vi "Rotating Ring.vi"(8 "error in (no error)":errorcluster, 11 "[V] Login in":refnum<class "[V] Login.lvclass">) -> (0 "error out":errorcluster, 3 "[V] Login out":refnum<class "[V] Login.lvclass">)   [LabVIEW 2020, in "[V] Login.lvlib" / "[V] Login.lvclass"]
uses:
  [V] Login.lvclass
  <vilib>/Analysis/NI_AALBase.lvlib
  <vilib>/Analysis/1siggen.llb/Ramp Pattern by Samples.vi
  <vilib>/picture/picture.llb/Draw True-Color Pixmap.vi
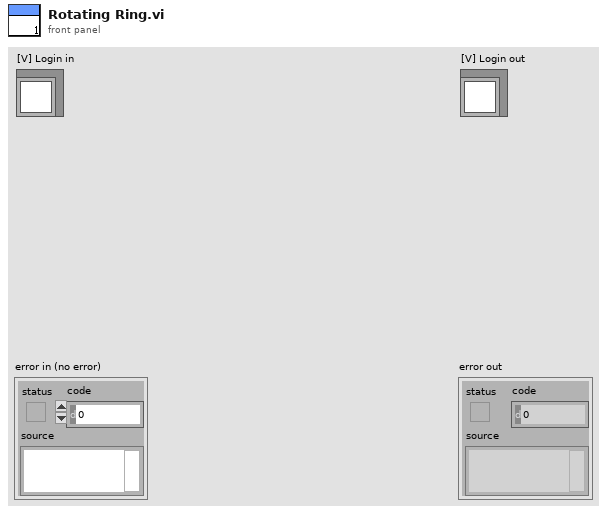
[diagram p1: front panel]
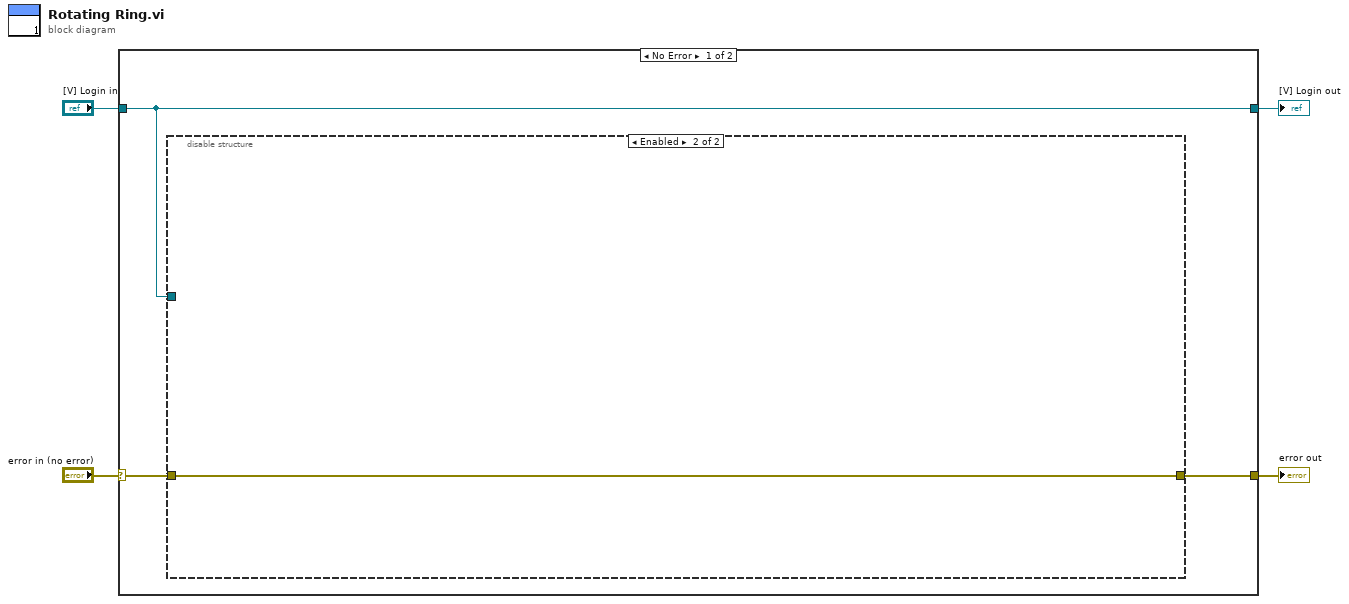
[diagram p0: block diagram]
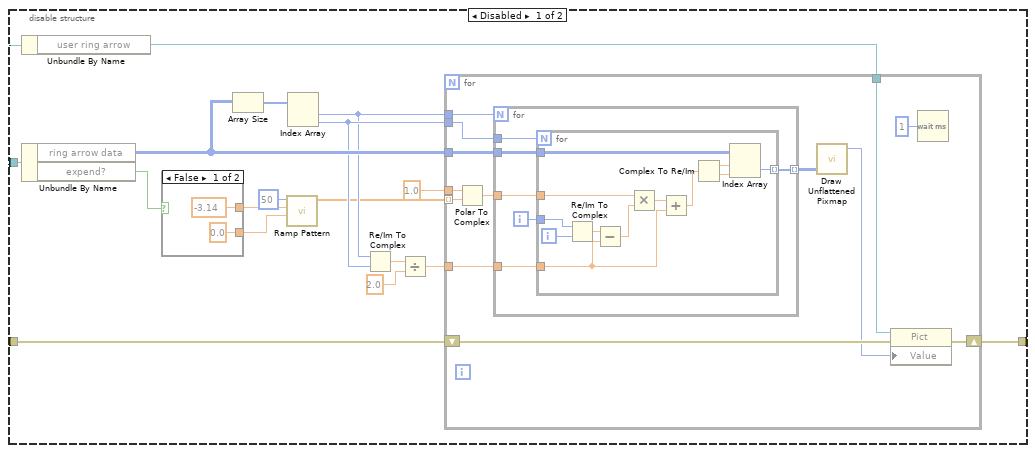
[diagram p2: hidden frame]
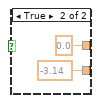
[diagram p3: hidden frame]
diagram:
  n1 = case shown="No Error" "error in (no error)" {
    selector: "error in (no error)" -> [w7 w62]
    tunnel: [w6 w62] -> w3
    tunnel: [w5 w61] -> w1
    tunnel: "[V] Login in" -> [w5 w61]
    frame No Error {
      n2 = disable-structure shown="Enabled" {
        disable-tunnel: w7 -> [w19 w60]
        disable-tunnel: [w16 w60] -> w6
        disable-tunnel: w5 -> [w8 _]
        frame Disabled {
          n3 = Unbundle By Name(w8) -> ("user ring arrow"=w18:refnum<vi>)
          n4 = Unbundle By Name(w8) -> ("ring arrow data"=w21:u32[][], "expend?"=w14:bool)
          n5 = case shown="False" w14 {
            tunnel: [-3.14 ("t") 0.0 ("t")] -> w13
            tunnel: [0.0 ("t") -3.14 ("t")] -> w10
            frame False {
            }
            frame True {
            }
          }
          n6 = Array Size(array=w21) -> (size(s)=w23:i32[])
          n7 = call-poly <vilib>:"Ramp Pattern.vi"("start"=w10, "end"=w13, "samples"=50) -> ("Ramp Pattern"=w11:dbl[])  [unwired: 7 in, 1 out]
          n8 = Index Array(array=w23) -> (element #1=w15:i32, element #2=w17:i32)  [unwired: 2 in]
          n9 = Re/Im To Complex(1:w17, 2:w15) -> (0:w24:cdb)
          n10 = Divide(x=w24, y=2.0) -> (x/y=w20:cdb)
          n11 = for {
            tunnel: w21 -> [w40]
            tunnel: w20 -> [w39]
            shift-right: [w36] -> w16
            shift-left: w19 -> [w37]
            tunnel: w18 -> [w35]
            tunnel: w17 -> [w33]
            tunnel: w11 -> [w32] mode=indexing
            tunnel: w15 -> [w31]
            tunnel: 1.0 ("r") -> [w30]
            n12 = Polar To Complex(1:w32, 2:w30) -> (0:w38:cdb)
            n13 = for {
              N: w31 -> [_]
              tunnel: w33 -> [w46]
              tunnel: w40 -> [w45]
              tunnel: [w44] -> w41 mode=indexing
              tunnel: w38 -> [w43]
              tunnel: w39 -> [w42]
              i -> [w47]
              n14 = for {
                N: w46 -> [_]
                tunnel: w47 -> [w56]
                tunnel: w45 -> [w59]
                tunnel: [w58] -> w44 mode=indexing
                tunnel: w43 -> [w53]
                tunnel: w42 -> [w48]
                i -> [w57]
                n15 = Re/Im To Complex(1:w57, 2:w56) -> (0:w55:cdb)
                n16 = Subtract(x=w55, y=w48) -> (x-y=w54:cdb)
                n17 = Multiply(x=w53, y=w54) -> (x*y=w52:cdb)
                n18 = Add(x=w52, y=w48) -> (x+y=w51:cdb)
                n19 = Complex To Re/Im(x + iy=w51) -> (x=w50:dbl, y=w49:dbl)
                n20 = Index Array(array=w59, index (row)=w50, index (col)=w49) -> (element=w58:u32)
              }
            }
            n21 = call-poly <vilib>:"Draw Unflattened Pixmap.vi"("data (RGB format)"=w41) -> ("new picture"=w34:picture)  [unwired: 8 in]
            n22 = property class="Pict"(reference=w35, error in=w37, "Value"=w34) -> (error out=w36:errorcluster)  [unwired: 1 out]
            n23 = Wait (ms)(milliseconds to wait=u32 1) -> ()  [unwired: 1 out]
          }
        }
        frame Enabled {
        }
      }
    }
    frame Error {
    }
  }
  "error out" <- w3
  "[V] Login out" <- w1
